vi "Do_Loop_Triggers.vi"(0 "Board ID":T3=1 min=1 max=32 step=1, 1 "Axis":T1=1 items=["Axis 1"=1, "Axis 2"=2, "Axis 3"=3, "Axis 4"=4, "Axis 5"=5, "Axis 6"=6, "Axis 7"=7, "Axis 8"=8], 2 "Reverse ?":bool, 5 "Number of steps":i32=10, 7 "Program (1)":T2=1 format="%.0x", 11 "error in (no error)":errorcluster, 12 "Total steps":i32, 13 "Offset":i32) -> (4 "Start Position":i32, 15 "error out":errorcluster)   [LabVIEW 2022 SP3]
doc: "EXAMPLE: DO_WHILE Loop (Onboard Programming Template)\n\nSUMMARY:\nThis FlexMotion example demonstrates the implementation of a DO_WHILE loop data structure in an onboard program. The C equivalent of the data structure implemented here is:\n\ndo {\n// code to be repeated\nloopVar = loopVar - increment;\n} while (loopVar != 0);\n\nTHEORY OF OPERATION:\nThe flow of the DO_WHILE loop data structure goes as follows:\n(1) Program storage is begun.\n(2) The DO_WHILE loop is set up. (Loop Variable and Increment are each defined and initialized.)\n(3) A code delimiter is set using label #1.\n(4) Code to be executed each time through loop is run (in the template program, the loop variable is decremented).\n(5) The loop variable or other test condition is checked.\n(6) If the test condition is true, then we jump back to label #1. Otherwise, the condition is false so the loop terminates.\n(7) Program storage is ended.\n\nDEVELOPMENT DETAILS:\nApplication Software: LabVIEW 5.0.x\nHardware: FlexMotion controller\nDriver Software: FlexMotion Software 4.0\n\nREQUIRED HARDWARE:\n(controller only)\n\nINSTRUCTIONS:\n(0) Initialize the FlexMotion controller before running this VI. \n(1) Add the FlexMotion functions you want to execute into the block diagram where noted.\n(2) Run the VI to store the program. (The program will not be executed at this time.)\n(3) You can then run the program you have stored by calling the run_prog.flx function with the appropriate program number.\n\nADDITIONAL NOTES:\n(a) You should read the following items before writing FlexMotion onboard programs:\n(1) The Onboard Programs section of the FlexMotion Hardware User Manual (page 4-9 in the November 1998 edition).\n(2) The section about onboard variables in your FlexMotion Software Reference Manual (pages 4-11 and 4-12 in the November 1998 edition)\n(3) You will find the chapter of the FlexMotion Software Reference Manual concerning the Onboard Programming functions to be an invaluable reference resource (Chapter 12 of the November 1998 edition) along with the online help for the VI functions.\n(b) This template repeats the DO_WHILE loop as long as an expression with a variable evaluates to be true. However, you may evaluate other conditions such as move complete status instead.\n\n*NOTE: This example is not supported on the 7334 controller."
uses:
  <vilib>/Motion/FlexMotion/FunctionsVIs/AnalogDigitalIO.llb/Set I/O Port MOMO.flx
  -MotionRoutines/MotionGlobals.vi
  <vilib>/Motion/FlexMotion/FunctionsVIs/AnalogDigitalIO.llb/Set I/O Port Direction.flx
  <vilib>/Motion/FlexMotion/FunctionsVIs/StartStopMotion.llb/Start Motion (8 axes).flx
  <vilib>/Motion/FlexMotion/FunctionsVIs/OnboardProgramming.llb/Jump to Label on Condition (8 axes).flx
  <vilib>/Motion/FlexMotion/FunctionsVIs/Trajectory.llb/Load Acceleration/Deceleration.flx
  <vilib>/Motion/FlexMotion/CustomControls/CustomControls.llb/Program.flx
  <vilib>/Motion/FlexMotion/CustomControls/CustomControls.llb/Axis To Read.flx
panel:
  out "Store Loop":i32
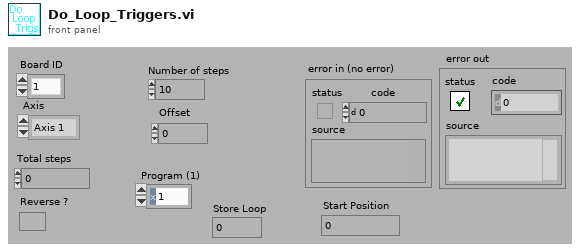
[diagram p1: front panel]
types:
  T1 = typedef "Axis To Read.flx" = u16
  T2 = typedef "Program.flx" = u8
  T3 = typedef "Board Id" = u8
  T4 = typedef "Var" = u8
  T5 = enum16{"Less Than", "Equal", "Less Than Or Equal", "Greater Than", "Not Equal", "Greater Than Or Equal", "True", "Home Found", "Index Found", "High Speed Capture", "Position Breakpoint", "Reserved", "Velocity Threshold", "Move Complete", "Profile Complete", "Blend Complete", "Motor Off", "Home Input Active", "Limit Input Active", "Software Limit Active", "Program Complete", "IO Port Match"}
  T6 = typedef "Bd Id Out" = u8
  T7 = typedef "MustOn" = cluster{"0":bool, "1":bool, "2":bool, "3":bool, "4":bool, "5":bool, "6":bool, "7":bool}
  T8 = typedef "Resource Out (Enum).flx" = u16
  T9 = cluster{"0":bool, "1":bool, "2":bool, "3":bool, "4":bool, "5":bool, "6":bool, "7":bool}
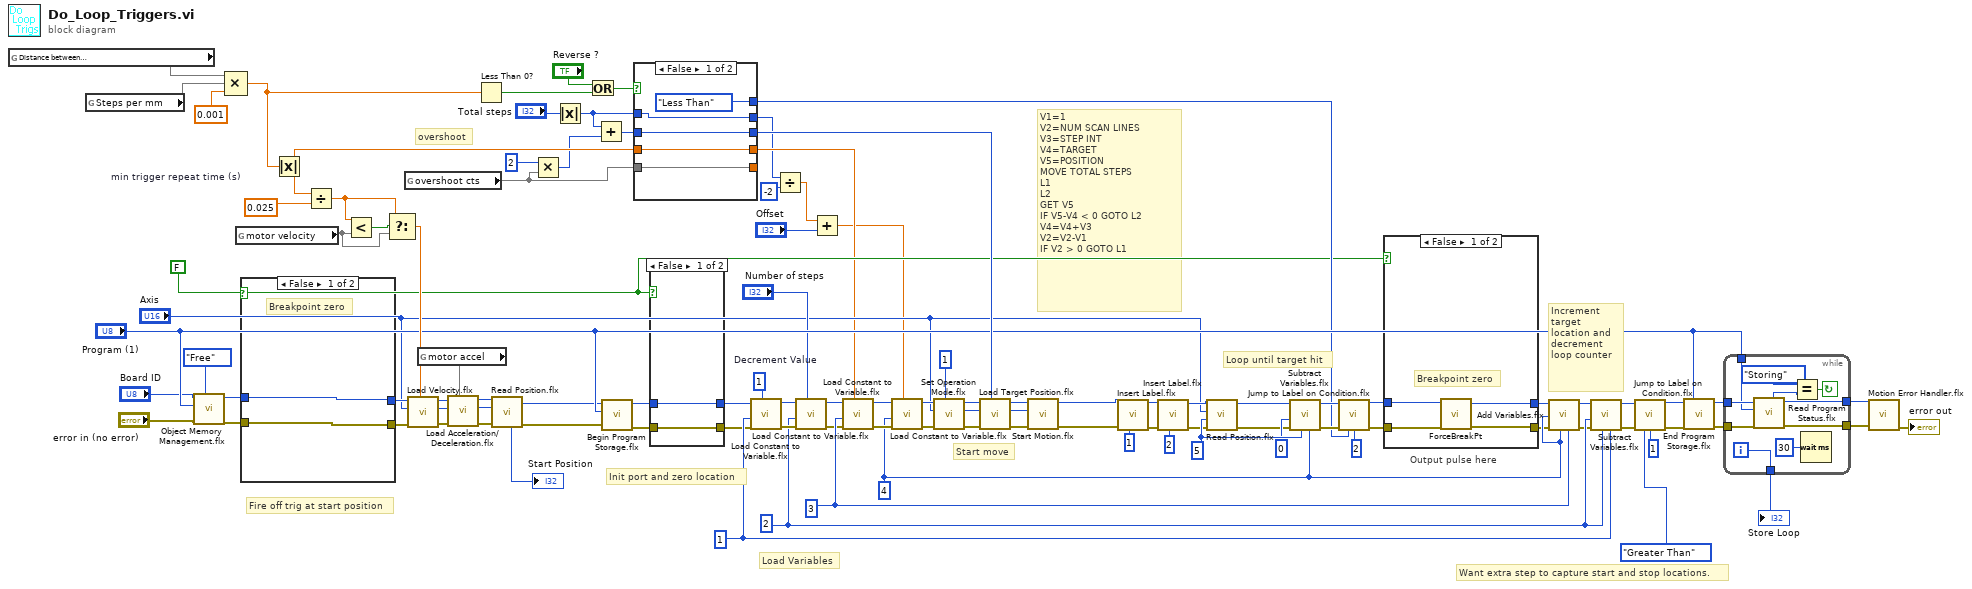
[diagram p0: block diagram]
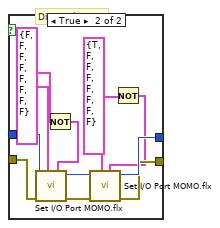
[diagram p2: hidden frame]
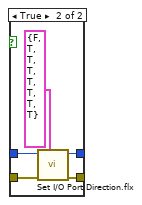
[diagram p3: hidden frame]
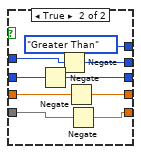
[diagram p4: hidden frame]
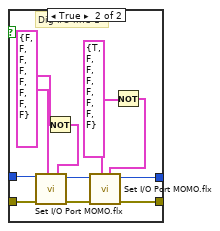
[diagram p5: hidden frame]
diagram:
  w24 = FALSE ("Case Constant\n(See Context Help)")
  w48 = 0.025  # min trigger repeat time (s)
  w85 = T4 4 ("Step Int Variable")
  w89 = T4 5 ("Position Variable")
  w86 = T4 3 ("Step Int Variable")
  w94 = T4 2 ("Loop Variable")
  w95 = T4 1 ("Decrement Variable")
  w96 = 1  # Decrement Value
  # "overshoot"
  # "Fire off trig at start position"
  # "V1=1\nV2=NUM SCAN LINES\nV3=STEP INT\nV4=TARGET\nV5=POSITION\nMOVE TOTAL STEPS\nL1\nL2\nGET V5\nIF V5-V4 < 0 GOTO L2\nV4=V4+V3\nV2=V2-V1\nIF V2 > 0 GOTO L1"
  # "Init port and zero location"
  # "Load Variables"
  # "Start move"
  # "Increment target location and decrement loop counter"
  # "Loop until target hit"
  # "Want extra step to capture start and stop locations."
  # "Output pulse here"
  n1 = global read "MotionGlobals.vi" "Distance between\nscan lines (mm)"() -> (w2)
  n2 = global read "MotionGlobals.vi" "Steps per mm"() -> (w4)
  n3 = call <vilib>:"Object Memory Management.flx"("Operation"=enum16{"Save", "Delete", "Free"}."Free" ("Operation (Free)"), "error in (no error)"="error in (no error)", "Object (1)"="Program (1)", "Board ID"="Board ID") -> ("error out"=w28:errorcluster, "Bd ID Out"=w25:T6)  [unwired: 4 out]
  n4 = Compound Arithmetic op=MULTIPLY(w2, w4, 0.001) -> (w1:dbl)
  n5 = global read "MotionGlobals.vi" "motor velocity"() -> (w38)
  n6 = case shown="False" w24 {
    tunnel: [w107 w115] -> w26
    tunnel: [w106 w114] -> w27
    tunnel: w25 -> [w107 w110]
    tunnel: w28 -> [w106 w112]
    frame False {
      # "Breakpoint zero"
    }
    frame True {
      w116 = T7 {"0"=TRUE, "1"=FALSE, "2"=FALSE, "3"=FALSE, "4"=FALSE, "5"=FALSE, "6"=FALSE, "7"=FALSE} ("Must On")
      w117 = T7 {"0"=FALSE, "1"=FALSE, "2"=FALSE, "3"=FALSE, "4"=FALSE, "5"=FALSE, "6"=FALSE, "7"=FALSE} ("Must On")
      # "Dig I/O line 1"
      n7 = Not(x=w117) -> (.not. x?=w109:T7)
      n8 = call "Set I/O Port MOMO.flx"("Must Off"=w109, "Must On"=w117, "error in (no error)"=w112, "Board ID"=w110) -> ("error out"=w113:errorcluster, "Bd ID Out"=w111:T6)  [unwired: 2 in, 2 out]
      n9 = Not(x=w116) -> (.not. x?=w108:T7)
      n10 = call "Set I/O Port MOMO.flx"("Must Off"=w108, "Must On"=w116, "error in (no error)"=w113, "Board ID"=w111) -> ("error out"=w114:errorcluster, "Bd ID Out"=w115:T6)  [unwired: 2 in, 2 out]
    }
  }
  n11 = Absolute Value(x=w1) -> (abs(x)=w39:dbl)
  n12 = Divide(x=w39, y=w48) -> (x/y=w46:dbl)
  n13 = Less?(x=w46, y=w38) -> (x < y?=w47:bool)
  n14 = Select(t=w46, s=w47, f=w38) -> (s? t:f=w45:dbl)
  n15 = global read "MotionGlobals.vi" "overshoot cts"() -> (w18)
  n16 = call <vilib>:"Load Velocity.flx"("Velocity (10000)"=w45, "error in (no error)"=w27, "Axis or Vector Space"="Axis", "Board ID"=w26) -> ("error out"=w35:errorcluster, "Resource Output"=w32:T8, "Bd ID Out"=w34:T6)  [unwired: 3 out]
  n17 = global read "MotionGlobals.vi" "motor accel"() -> (w33)
  n18 = call "Load Acceleration/Deceleration.flx"("Acceleration (100000)"=w33, "error in (no error)"=w35, "Axis or Vector Space"=w32, "Board ID"=w34) -> ("error out"=w36:errorcluster, "Resource Output"=w29:T8, "Bd ID Out"=w37:T6)  [unwired: 1 in, 2 out]
  n19 = Less Than 0?(x=w1) -> (x < 0?=w42:bool)
  n20 = call <vilib>:"Read Position.flx"("error in (no error)"=w36, "Axis"=w29, "Board ID"=w37) -> ("error out"=w12:errorcluster, "Bd ID Out"=w13:T6, "Position"=→"Start Position":i32)  [unwired: 4 out]
  n21 = Multiply(x=2, y=w18) -> (x*y=w20:i32)
  n22 = Absolute Value(x="Total steps") -> (abs(x)=w11:i32)
  n23 = Or(x="Reverse ?", y=w42) -> (x .or. y?=w40:bool)
  n24 = Add(x=w11, y=w20) -> (x+y=w22:i32)
  n25 = call <vilib>:"Begin Program Storage.flx"("error in (no error)"=w12, "Program (1)"="Program (1)", "Board ID"=w13) -> ("error out"=w83:errorcluster, "Bd ID Out"=w82:T6)  [unwired: 4 out]
  n26 = case shown="False" w40 {
    tunnel: w22 -> [w122 w131]
    tunnel: [w122 w130] -> w50
    tunnel: [w121 w128] -> w10
    tunnel: w39 -> [w121 w129]
    tunnel: [T5."Less Than" ("Condition Code (True)") T5."Greater Than" ("Condition Code (True)")] -> w43
    tunnel: [w119 w125] -> _
    tunnel: w18 -> [w119 w126]
    tunnel: w11 -> [w118 w124]
    tunnel: [w118 w123] -> w9
    frame False {
    }
    frame True {
      n27 = Negate(x=w131) -> (-x=w130:i32)
      n28 = Negate(x=w124) -> (-x=w123:i32)
      n29 = Negate(x=w129) -> (-x=w128:dbl)
      n30 = Negate(x=w126) -> (-x=w125:dbl)
    }
  }
  n31 = case shown="False" w24 {
    tunnel: w83 -> [w132 w138]
    tunnel: w82 -> [w133 w137]
    tunnel: [w133 w135] -> w59
    tunnel: [w132 w134] -> w58
    frame False {
    }
    frame True {
      n32 = call "Set I/O Port Direction.flx"("Direction (Input)"=T9 {"0"=FALSE, "1"=TRUE, "2"=TRUE, "3"=TRUE, "4"=TRUE, "5"=TRUE, "6"=TRUE, "7"=TRUE}, "error in (no error)"=w138, "Board ID"=w137) -> ("error out"=w134:errorcluster, "Bd ID Out"=w135:T6)  [unwired: 1 in, 4 out]
    }
  }
  n33 = call <vilib>:"Load Constant to Variable.flx"("Value (0)"=w96, "error in (no error)"=w58, "Var"=w95, "Board ID"=w59) -> ("error out"=w99:errorcluster, "Bd ID Out"=w101:T6)  [unwired: 4 out]
  n34 = Divide(x=w9, y=-2) -> (x/y=w16:dbl)
  n35 = call <vilib>:"Load Constant to Variable.flx"("Value (0)"="Number of steps", "error in (no error)"=w99, "Var"=w94, "Board ID"=w101) -> ("error out"=w80:errorcluster, "Bd ID Out"=w81:T6)  [unwired: 4 out]
  n36 = Add(x=w16, y="Offset") -> (x+y=w8:dbl)
  n37 = call <vilib>:"Load Constant to Variable.flx"("Value (0)"=w10, "error in (no error)"=w80, "Var"=w86, "Board ID"=w81) -> ("error out"=w87:errorcluster, "Bd ID Out"=w88:T6)  [unwired: 4 out]
  n38 = call <vilib>:"Load Constant to Variable.flx"("Value (0)"=w8, "error in (no error)"=w87, "Var"=w85, "Board ID"=w88) -> ("error out"=w64:errorcluster, "Bd ID Out"=w65:T6)  [unwired: 4 out]
  n39 = call <vilib>:"Set Operation Mode.flx"("Position Mode (Absolute)"=1, "error in (no error)"=w64, "Axis or Vector Space"="Axis", "Board ID"=w65) -> ("error out"=w62:errorcluster, "Resource Output"=w57:T8, "Bd ID Out"=w63:T6)  [unwired: 2 out]
  n40 = call <vilib>:"Load Target Position.flx"("Target Position (0)"=w50, "error in (no error)"=w62, "Axis"=w57, "Board ID"=w63) -> ("error out"=w66:errorcluster, "Resource Output"=w67:T8, "Bd ID Out"=w60:T6)  [unwired: 3 out]
  n41 = call-poly <vilib>:"Start Motion.flx"("error in (no error)"=w66, "Axis or Vector Space"=w67, "Board ID"=w60) -> ("error out"=w55:errorcluster, "Bd ID Out"=w56:T6)  [unwired: 1 in, 3 out]
  n42 = call <vilib>:"Insert Label.flx"("Label Number (1)"=u16 1 ("Label"), "error in (no error)"=w55, "Board ID"=w56) -> ("error out"=w78:errorcluster, "Bd ID Out"=w79:T6)  [unwired: 4 out]
  n43 = call <vilib>:"Insert Label.flx"("Label Number (1)"=u16 2 ("Label"), "error in (no error)"=w78, "Board ID"=w79) -> ("error out"=w76:errorcluster, "Bd ID Out"=w77:T6)  [unwired: 4 out]
  n44 = call <vilib>:"Read Position.flx"("error in (no error)"=w76, "Retn Vect"=w89, "Axis"="Axis", "Board ID"=w77) -> ("error out"=w74:errorcluster, "Bd ID Out"=w75:T6)  [unwired: 4 out]
  n45 = call <vilib>:"Subtract Variables.flx"("Var 2"=w85, "Var 1"=w89, "error in (no error)"=w74, "Ret Vect"=T4 0 ("Position Variable"), "Board ID"=w75) -> ("error out"=w72:errorcluster, "Bd ID Out"=w73:T6)  [unwired: 3 out]
  n46 = call-poly <vilib>:"Jump to Label on Condition.flx"("Board ID"=w73, "error in (no error)"=w72, "Condition Code (True)"=w43, "Jump to Label (1)"=u16 2) -> ("Bd ID Out"=w69:T6, "error out"=w68:errorcluster)  [unwired: 4 in, 6 out]
  n47 = case shown="False" w24 {
    tunnel: [w142 w150] -> w71
    tunnel: [w141 w149] -> w70
    tunnel: w69 -> [w140 w145]
    tunnel: w68 -> [w139 w147]
    frame False {
      # "Breakpoint zero"
      n48 = call "ForceBreakPt.vi"("error in"=w139, "Bd ID in"=w140) -> ("error out"=w141:errorcluster, "Bd ID Out"=w142:u8)
    }
    frame True {
      w151 = T7 {"0"=TRUE, "1"=FALSE, "2"=FALSE, "3"=FALSE, "4"=FALSE, "5"=FALSE, "6"=FALSE, "7"=FALSE} ("Must On")
      w152 = T7 {"0"=FALSE, "1"=FALSE, "2"=FALSE, "3"=FALSE, "4"=FALSE, "5"=FALSE, "6"=FALSE, "7"=FALSE} ("Must On")
      # "Dig I/O line 1"
      n49 = Not(x=w152) -> (.not. x?=w144:T7)
      n50 = call "Set I/O Port MOMO.flx"("Must Off"=w144, "Must On"=w152, "error in (no error)"=w147, "Board ID"=w145) -> ("error out"=w148:errorcluster, "Bd ID Out"=w146:T6)  [unwired: 2 in, 2 out]
      n51 = Not(x=w151) -> (.not. x?=w143:T7)
      n52 = call "Set I/O Port MOMO.flx"("Must Off"=w143, "Must On"=w151, "error in (no error)"=w148, "Board ID"=w146) -> ("error out"=w149:errorcluster, "Bd ID Out"=w150:T6)  [unwired: 2 in, 2 out]
    }
  }
  n53 = call <vilib>:"Add Variables.flx"("Var 2"=w86, "Var 1"=w85, "error in (no error)"=w70, "Ret Vect"=w85, "Board ID"=w71) -> ("error out"=w91:errorcluster, "Bd ID Out"=w90:T6)  [unwired: 3 out]
  n54 = call <vilib>:"Subtract Variables.flx"("Var 2"=w95, "Var 1"=w94, "error in (no error)"=w91, "Ret Vect"=w94, "Board ID"=w90) -> ("error out"=w97:errorcluster, "Bd ID Out"=w100:T6)  [unwired: 3 out]
  n55 = call-poly <vilib>:"Jump to Label on Condition.flx"("Board ID"=w100, "error in (no error)"=w97, "Condition Code (True)"=T5."Greater Than", "Jump to Label (1)"=u16 1) -> ("Bd ID Out"=w104:T6, "error out"=w98:errorcluster)  [unwired: 4 in, 6 out]
  n56 = call <vilib>:"End Program Storage.flx"("error in (no error)"=w98, "Program (1)"="Program (1)", "Board ID"=w104) -> ("error out"=w52:errorcluster, "Bd ID Out"=w53:T6)  [unwired: 4 out]
  n57 = while {
    tunnel: w53 -> [w162]
    tunnel: w52 -> [w161]
    tunnel: [w160] -> w7
    tunnel: [w159] -> w6
    tunnel: "Program (1)" -> [w158]
    tunnel: [w154] -> w51
    i -> [w154]
    stop <- w155 continue-if-true
    n58 = call <vilib>:"Read Program Status.flx"("error in (no error)"=w161, "Program (1)"=w158, "Board Id"=w162) -> ("error out"=w159:errorcluster, "Bd Id Out"=w160:T6, "Program Status"=w156:enum16{"Done", "Playing", "Paused", "Storing"})  [unwired: 4 out]
    n59 = Equal?(x=enum16{"Done", "Playing", "Paused", "Storing"}."Storing" ("Program Status"), y=w156) -> (x = y?=w155:bool)
    n60 = Wait (ms)(milliseconds to wait=30) -> ()  [unwired: 1 out]
  }
  "Store Loop" <- w51
  n61 = call <vilib>:"Motion Error Handler.flx"("Board ID"=w7, "error in (no error)"=w6) -> ("error out"=→"error out":errorcluster)  [unwired: 3 in, 10 out]
